vi "File.Archive Dir Mover.vi"(8 "TempLocal":path=path "C:/MTE/Data/ArchiveTemp", 9 "Error Msg":T1={"Cmd"="Task", "Sub"="Warning", "Data1"=variant, "Data2"=variant}, 10 "Parent Q":refnum<queue>, 11 "Q Name":string="FileMover") -> ()   [LabVIEW 2018]
uses:
  <vilib>/KATE/Queues/Q.Element.ctl
  Archive Mover/File.ArchiveMover Task.ctl
  <vilib>/KATE/Queues/Queue Utils.lvlib
  <vilib>/KATE/Scheduler/Scheduler.lvlib
  <vilib>/KATE/Files/File Utils.lvlib
  <vilib>/KATE/Status/Status Utils.lvlib
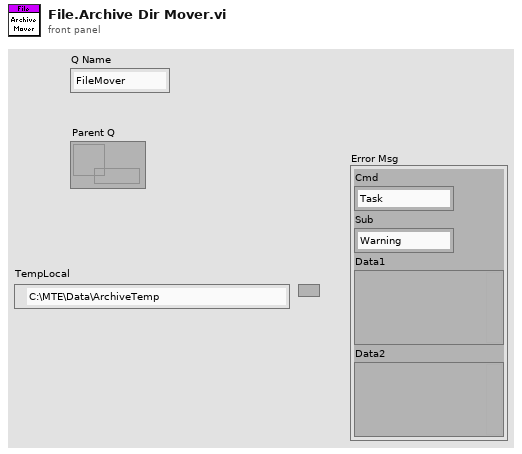
[diagram p1: front panel]
types:
  T1 = typedef "KATE_Lib.lvlib/Queue Utils.lvlib/Q.Element.ctl" = cluster{"Cmd":string, "Sub":string, "Data1":variant, "Data2":variant}
  T2 = typedef "File.ArchiveMover Task.ctl" = cluster{"Source":path, "DestDir":path, "New Name":string, "SubDirs":string[]}
  T3 = cluster{"TempDir":path, "ArchiveDir":path, "Task":T2}
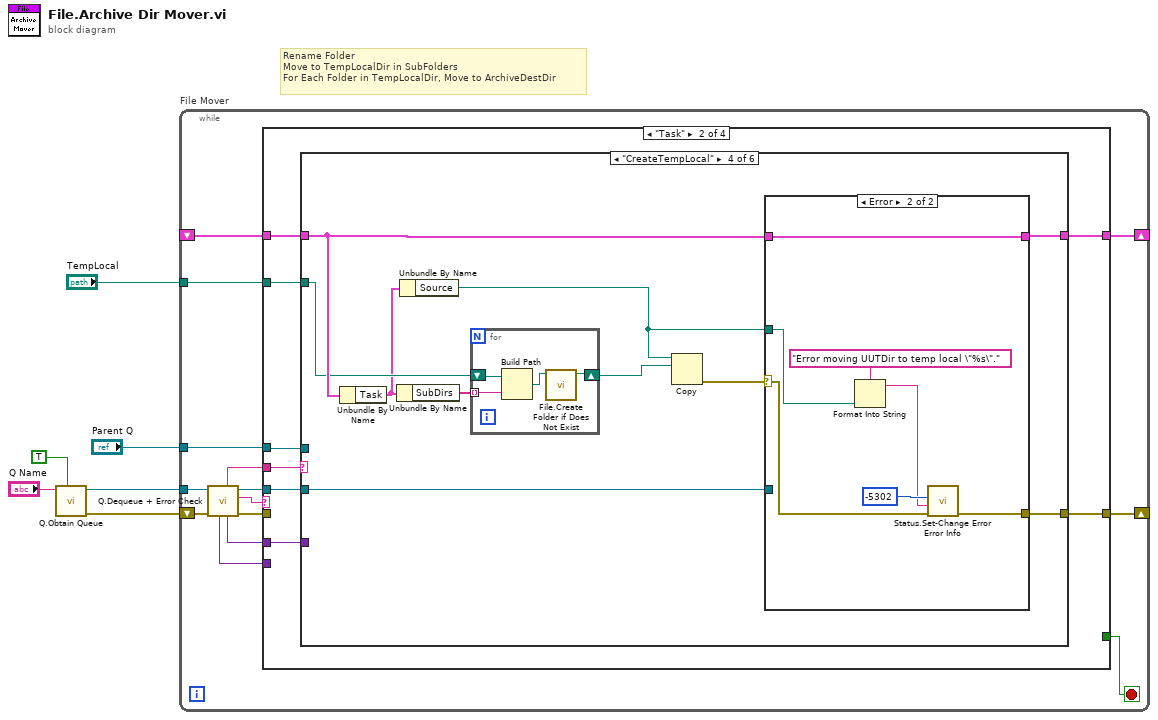
[diagram p0: block diagram]
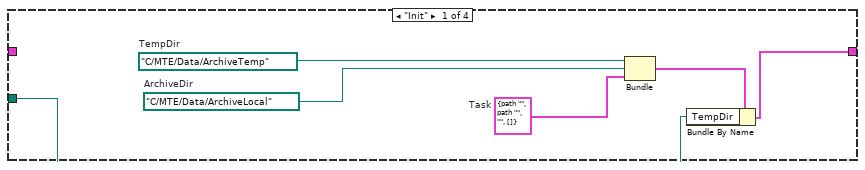
[diagram p2: hidden frame]
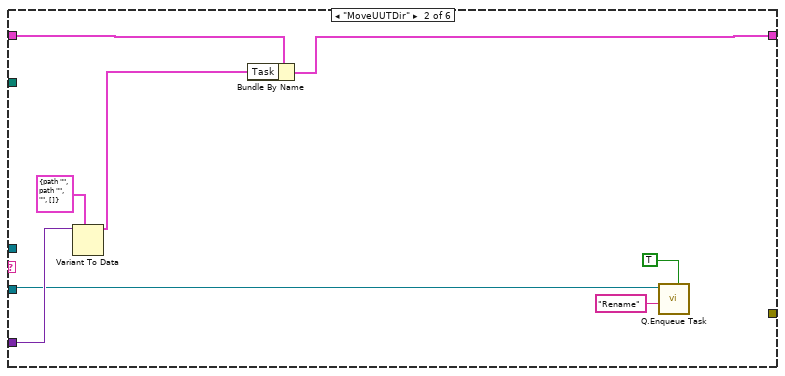
[diagram p4: hidden frame]
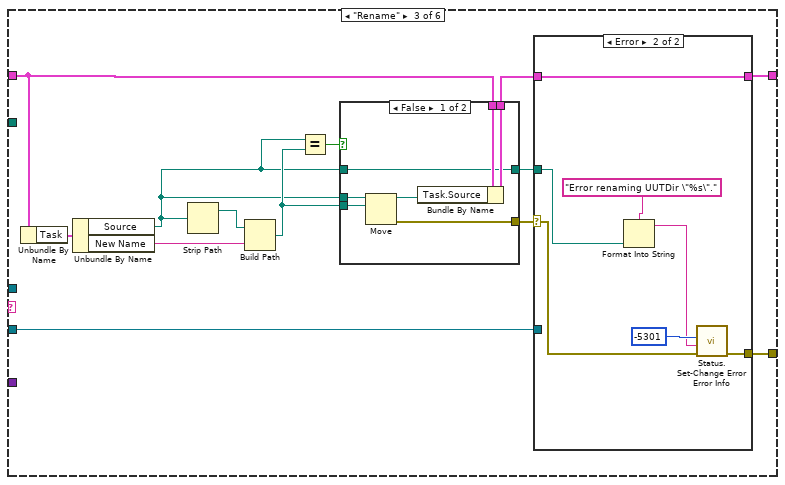
[diagram p5: hidden frame]
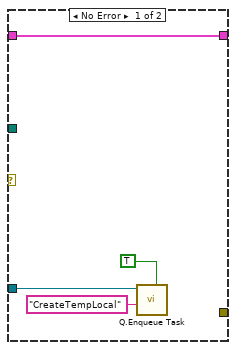
[diagram p7: hidden frame]
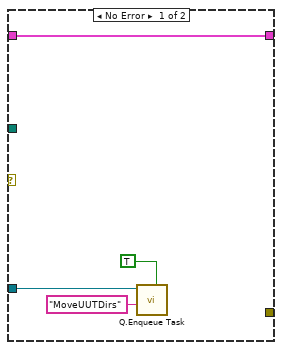
[diagram p8: hidden frame]
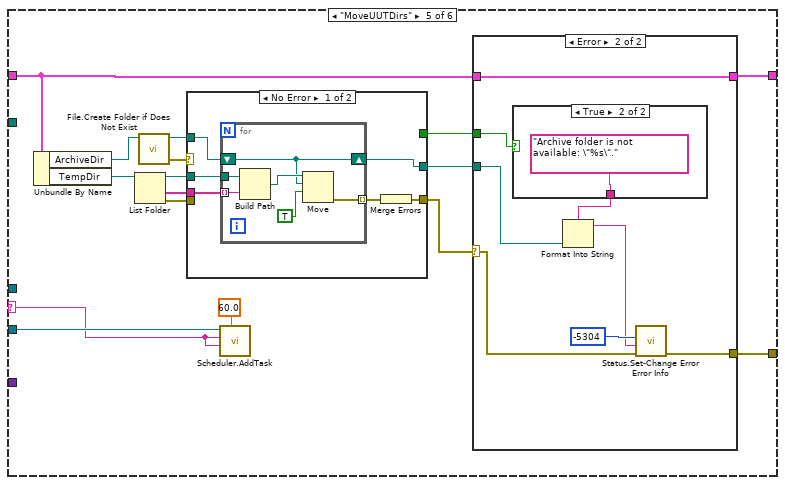
[diagram p9: hidden frame]
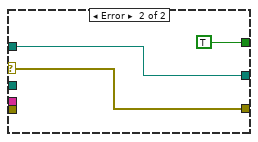
[diagram p10: hidden frame]
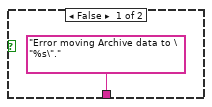
[diagram p12: hidden frame]
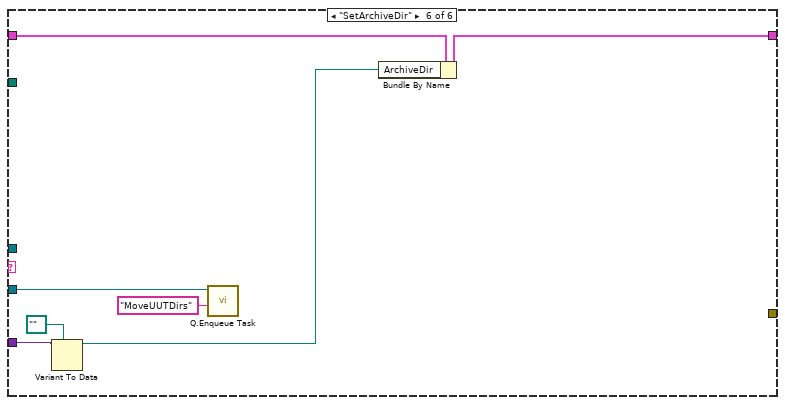
[diagram p13: hidden frame]
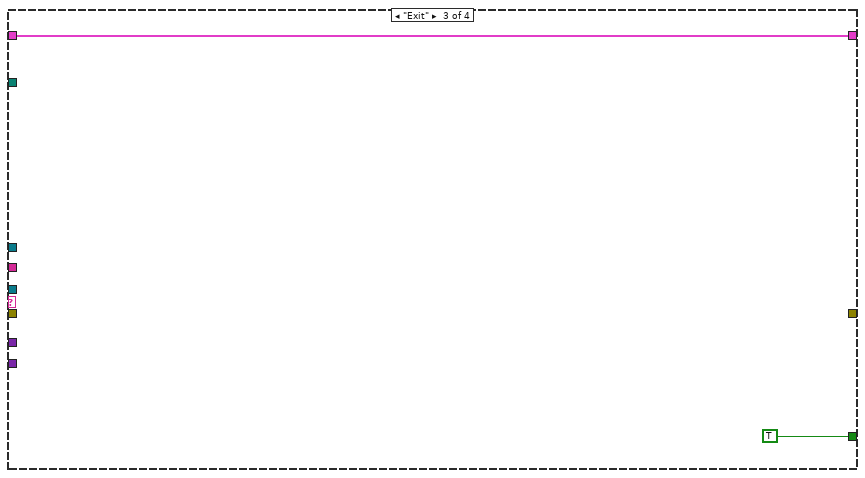
[diagram p14: hidden frame]
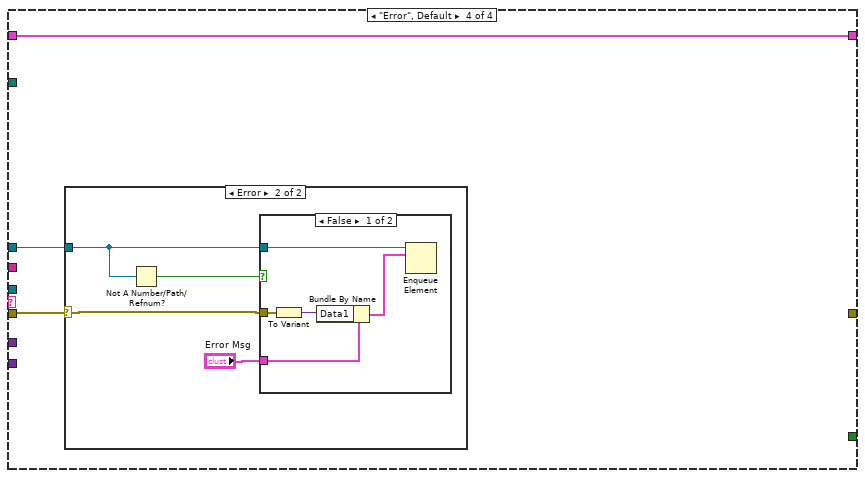
[diagram p15: hidden frame]
diagram:
  # "Rename Folder\nMove to TempLocalDir in SubFolders\nFor Each Folder in TempLocalDir, Move to ArchiveDestDir"
  n1 = call <vilib>:"Q.Obtain Queue.vi"("Enqueue Init"=TRUE, "Q Name"="Q Name") -> ("error out"=w6:errorcluster, "Q Out"=w5:refnum<queue>)  [unwired: 7 in, 1 out]
  n2 = while "File Mover" {
    tunnel: w5 -> [w20]
    shift-right: [w15] -> _
    shift-left: w6 -> [w19]
    tunnel: "Parent Q" -> [w13]
    shift-right: [w9] -> _
    shift-left: _ -> [w8]
    tunnel: "TempLocal" -> [w7]
    stop <- w12 stop-if-true
    n3 = call <vilib>:"Q.Dequeue + Error Check.vi"("Error In"=w19, "Q In"=w20) -> ("error out"=w11:errorcluster, "Cmd"=w14:string, "Q Out"=w18:refnum<queue>, "Data1"=w17:variant, "Sub"=w10:string, "Data2"=w16:variant)  [unwired: 4 in]
    n4 = case shown="\"Task\"" w14 {
      tunnel: w18 -> [_ w30 _ _]
      tunnel: w17 -> [_ w34 _ _]
      tunnel: w16 -> [_ _ _ _]
      tunnel: [_ w33 _ _] -> w15
      tunnel: w13 -> [_ w31 _ w154]
      tunnel: [_ _ TRUE _] -> w12
      tunnel: w11 -> [_ _ _ w155]
      tunnel: w10 -> [_ w32 _ _]
      tunnel: [w22 w28 w151 w153] -> w9
      tunnel: w8 -> [_ w29 w151 w153]
      tunnel: w7 -> [w21 w27 _ _]
      frame "Init" {
        w25 = T2 {"Source"=path "", "DestDir"=path "", "New Name"="", "SubDirs"=[]}  # Task
        w26 = path "C:/MTE/Data/ArchiveLocal"  # ArchiveDir
        w24 = path "C:/MTE/Data/ArchiveTemp"  # TempDir
        n5 = Bundle("TempDir"=w24, "ArchiveDir"=w26, "Task"=w25) -> (w23:T3)  [unwired: 1 in]
        n6 = Bundle By Name(cluster=w23, "TempDir"=w21) -> (w22:T3)
      }
      frame "Task" {
        n7 = case shown="\"CreateTempLocal\"" w32 {
          selector: w32 -> [_ _ _ _ w105 _]
          tunnel: w34 -> [_ w43 _ _ _ w150]
          tunnel: [_ _ w55 w85 w116 _] -> w33
          tunnel: w31 -> [_ _ _ _ _ _]
          tunnel: w30 -> [_ w37 w44 w77 w106 w144]
          tunnel: w29 -> [w35 w40 w49 w83 w115 w146]
          tunnel: [w35 w42 w56 w86 w117 w147] -> w28
          tunnel: w27 -> [_ _ _ w81 _ _]
          frame Default {
          }
          frame "MoveUUTDir" {
            n8 = Variant To Data(type=T2 {"Source"=path "", "DestDir"=path "", "New Name"="", "SubDirs"=[]} ("output cluster"), Variant=w43) -> (data=w39:T2)  [unwired: 1 in, 1 out]
            n9 = Bundle By Name(cluster=w40, "Task"=w39) -> (w42:T3)
            n10 = call <vilib>:"Q.Enqueue Task.vi"("Top of Q"=TRUE, "Task Name"="Rename", "Q In"=w37) -> ()  [unwired: 7 in, 2 out]
          }
          frame "Rename" {
            n11 = Unbundle By Name(w49) -> ("Task"=w51:T2)
            n12 = Unbundle By Name(w51) -> ("Source"=w46:path, "New Name"=w54:string)
            n13 = Strip Path(path=w46) -> (stripped path=w53:path)  [unwired: 1 out]
            n14 = Build Path(base path=w53, name or relative path=w54) -> (appended path=w48:path)
            n15 = Equal?(x=w46, y=w48) -> (x = y?=w47:bool)
            n16 = case shown="False" w47 {
              tunnel: [w63 _] -> w52
              tunnel: [w62 w65] -> w50
              tunnel: w49 -> [w61 w65]
              tunnel: w48 -> [w59 _]
              tunnel: w46 -> [w58 _]
              tunnel: w46 -> [w57 w64]
              tunnel: [w57 w64] -> w45
              frame False {
                n17 = Move(source path=w58, 10:w59) -> (error out=w63:errorcluster, 3:w60:path)  [unwired: 3 in, 1 out]
                n18 = Bundle By Name(cluster=w61, "Task.Source"=w60) -> (w62:T3)
              }
              frame True {
              }
            }
            n19 = case shown="Error" w52 {
              selector: w52 -> [_ w70]
              tunnel: w50 -> [w69 w76]
              tunnel: [w69 w76] -> w56
              tunnel: [_ w75] -> w55
              tunnel: w44 -> [w68 _]
              tunnel: w45 -> [_ w72]
              frame No Error {
                n20 = call <vilib>:"Q.Enqueue Task.vi"("Top of Q"=TRUE, "Task Name"="CreateTempLocal", "Q In"=w68) -> ()  [unwired: 7 in, 2 out]
              }
              frame Error {
                n21 = Format Into String(format string="Error renaming UUTDir \"%s\".", w72) -> (resulting string=w71:string)  [unwired: 2 in, 1 out]
                n22 = call <vilib>:"Status.Set-Change Error Error Info.vi"("Error In"=w70, "NewDesc"=w71, "NewCode"=-5301) -> ("Error Out"=w75:errorcluster)  [unwired: 8 in]
              }
            }
          }
          frame "CreateTempLocal" {
            n23 = Unbundle By Name(w83) -> ("Task"=w80:T2)
            n24 = Unbundle By Name(w80) -> ("SubDirs"=w82:string[])
            n25 = Unbundle By Name(w80) -> ("Source"=w78:path)
            n26 = for {
              tunnel: w82 -> [w90] mode=indexing
              shift-right: [w87] -> w79
              shift-left: w81 -> [w89]
              n27 = Build Path(base path=w89, name or relative path=w90) -> (appended path=w88:path)
              n28 = call <vilib>:"File.Create Folder if Does Not Exist.vi"("Path"=w88) -> ("Dup Path"=w87:path)  [unwired: 8 in, 2 out]
            }
            n29 = Copy(10:w79, 11:w78) -> (0:w84:errorcluster)  [unwired: 3 in, 2 out]
            n30 = case shown="Error" w84 {
              selector: w84 -> [_ w95]
              tunnel: w83 -> [w94 w101]
              tunnel: [w94 w101] -> w86
              tunnel: [_ w100] -> w85
              tunnel: w77 -> [w93 _]
              tunnel: w78 -> [_ w97]
              frame No Error {
                n31 = call <vilib>:"Q.Enqueue Task.vi"("Top of Q"=TRUE, "Task Name"="MoveUUTDirs", "Q In"=w93) -> ()  [unwired: 7 in, 2 out]
              }
              frame Error {
                n32 = Format Into String(format string="Error moving UUTDir to temp local \"%s\".", w97) -> (resulting string=w96:string)  [unwired: 2 in, 1 out]
                n33 = call <vilib>:"Status.Set-Change Error Error Info.vi"("Error In"=w95, "NewDesc"=w96, "NewCode"=-5302) -> ("Error Out"=w100:errorcluster)  [unwired: 8 in]
              }
            }
          }
          frame "MoveUUTDirs" {
            n34 = Unbundle By Name(w115) -> ("ArchiveDir"=w109:path, "TempDir"=w114:path)
            n35 = List Folder(path=w114) -> (path out=w113:path, folder names=w112:string[], error out=w102:errorcluster)  [unwired: 3 in, 1 out]
            n36 = call <vilib>:"File.Create Folder if Does Not Exist.vi"("Path"=w109) -> ("error out"=w104:errorcluster, "Dup Path"=w108:path)  [unwired: 8 in, 1 out]
            n37 = case shown="No Error" w104 {
              selector: w104 -> [_ w131]
              tunnel: w113 -> [w123 _]
              tunnel: w112 -> [w122 _]
              tunnel: [w120 w131] -> w111
              tunnel: [w119 w132] -> w110
              tunnel: w108 -> [w118 w132]
              tunnel: [_ TRUE] -> w103
              tunnel: w102 -> [_ _]
              frame No Error {
                n38 = for {
                  tunnel: w123 -> [w128]
                  tunnel: w122 -> [w129] mode=indexing
                  tunnel: [w127] -> w121 mode=indexing
                  shift-right: [w125] -> w119
                  shift-left: w118 -> [w125]
                  n39 = Build Path(base path=w128, name or relative path=w129) -> (appended path=w126:path)
                  n40 = Move(source path=w126, 9:TRUE ("overwrite (F)"), 10:w125) -> (error out=w127:errorcluster)  [unwired: 2 in, 2 out]
                }
                n41 = Merge Errors(w121) -> (w120:errorcluster)
              }
              frame Error {
              }
            }
            n42 = call <vilib>:"Scheduler.AddTask.vi"("Interval(s)"=60.0, "Task Name"=w105, "Sched Name"=w105, "Q In"=w106) -> ()  [unwired: 6 in, 2 out]
            n43 = case shown="Error" w111 {
              selector: w111 -> [_ w135]
              tunnel: w115 -> [w133 w141]
              tunnel: [w133 w141] -> w117
              tunnel: [_ w140] -> w116
              tunnel: w110 -> [_ w137]
              tunnel: w103 -> [_ w134]
              frame No Error {
              }
              frame Error {
                n44 = case shown="True" w134 {
                  tunnel: ["Error moving Archive data to \"%s\"." "Archive folder is not available: \"%s\"."] -> w138
                  frame False {
                  }
                  frame True {
                  }
                }
                n45 = Format Into String(format string=w138, w137) -> (resulting string=w136:string)  [unwired: 2 in, 1 out]
                n46 = call <vilib>:"Status.Set-Change Error Error Info.vi"("Error In"=w135, "NewDesc"=w136, "NewCode"=-5304) -> ("Error Out"=w140:errorcluster)  [unwired: 8 in]
              }
            }
          }
          frame "SetArchiveDir" {
            n47 = Variant To Data(type=path "", Variant=w150) -> (data=w148:path)  [unwired: 1 in, 1 out]
            n48 = call <vilib>:"Q.Enqueue Task.vi"("Task Name"="MoveUUTDirs", "Q In"=w144) -> ()  [unwired: 8 in, 2 out]
            n49 = Bundle By Name(cluster=w146, "ArchiveDir"=w148) -> (w147:T3)
          }
        }
      }
      frame "Exit" {
        (unwired) TRUE
      }
      frame "Error", Default {
        n50 = case shown="Error" w155 {
          selector: w155 -> [_ w156]
          tunnel: w154 -> [_ w158]
          frame No Error {
          }
          frame Error {
            n51 = Not A Number/Path/Refnum?(number/path/refnum=w158) -> (NaN/Path/Refnum?=w159:bool)
            n52 = case shown="False" w159 {
              tunnel: w158 -> [w164 _]
              tunnel: "Error Msg" -> [w163 _]
              tunnel: w156 -> [w160 _]
              frame False {
                n53 = To Variant(anything=w160) -> (Variant=w161:variant)
                n54 = Bundle By Name(cluster=w163, "Data1"=w161) -> (w162:T1)
                n55 = Enqueue Element(queue=w164, element=w162) -> ()  [unwired: 2 in, 3 out]
              }
              frame True {
              }
            }
          }
        }
      }
    }
  }
